vi "6517A.vi"() -> ()   [LabVIEW 2019]
uses:
  lib/Keithley 622x/Configure/Delta PDelta DCon Modes/Low Level/Typedefs/KE622x -- Delta DCon Mode Delay.ctl
  <vilib>/Utility/file.llb/Write Delimited Spreadsheet (DBL).vi
  lib/Keithley 622x/Keithley 622x.lvlib
  lib/Keithley 6517/Keithley 6517.lvlib
panel:
  in  "I(A)":dbl
  out "XY图":cluster{dbl[], dbl[]}(graph)
  in  "file path (dialog if empty)":path caption="文件路径 （空时为对话框）"
  in  "622x Resource":refnum<visa-resource-name>
  in  "Meas Timeout\n(msecs)":u32=20000
  out "Execution Time\n(secs)":dbl
  in  "Instrument Type":i32(ring)=3 items=["PPMS", "VersaLab", "DynaCool", "SVSM"]
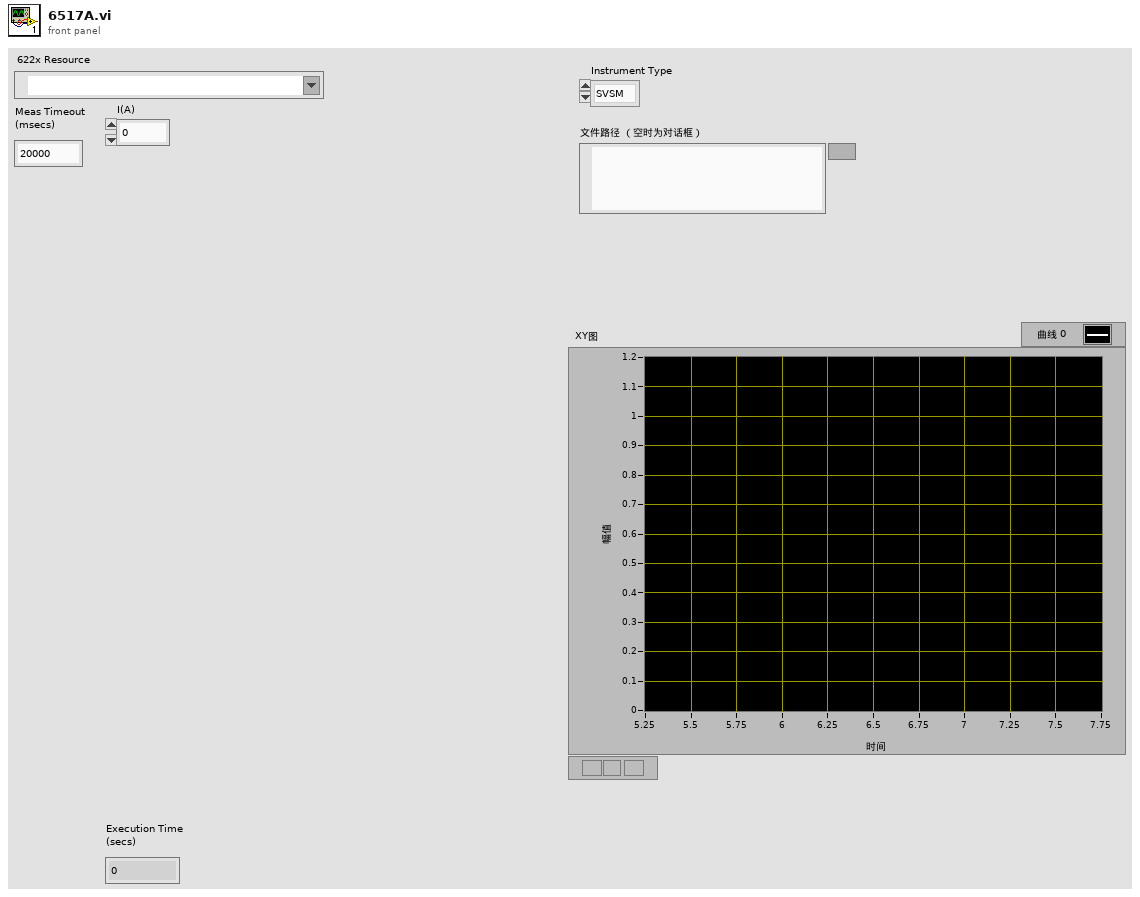
[diagram p1: front panel]
types:
  T1 = enum16{"open", "replace", "create", "open or create", "replace or create", "replace or create with confirmation"}
  T2 = typedef "Keithley 622x.lvlib/KE622x -- Delta DCon Mode Delay.ctl" = dbl
  T3 = cluster{"Measurement":dbl, "Units":string, "Time Stamp and Date":string, "Reading #":dbl, "Channel #":dbl}
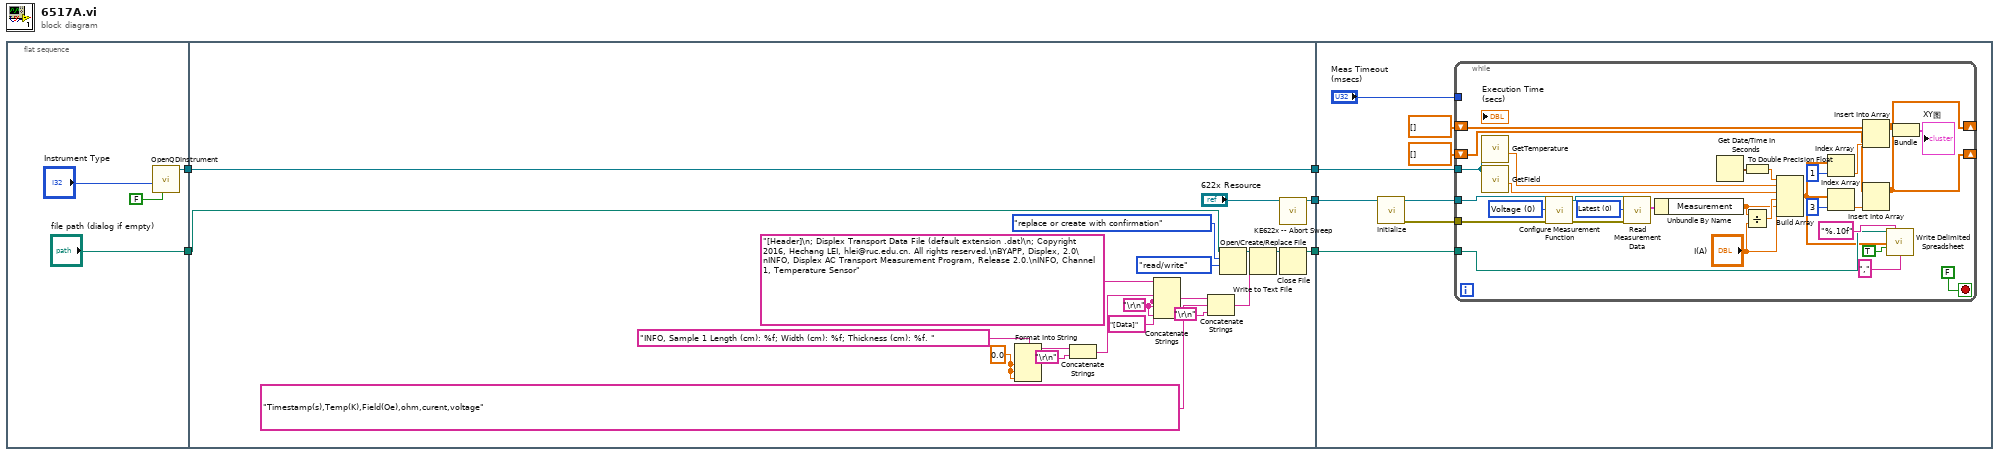
[diagram p0: block diagram]
diagram:
  n1 = flat-sequence {
    tunnel: [w7] -> w5
    tunnel: ["file path (dialog if empty)"] -> w3
    tunnel: w5 -> [w30]
    tunnel: [w30] -> w4
    tunnel: w3 -> [w18]
    tunnel: [w13] -> w2
    tunnel: [w10] -> w1
    tunnel: w4 -> [w38]
    tunnel: w2 -> [w36]
    tunnel: w1 -> [w33]
    frame #0 {
      n2 = call "OpenQDInstrument.vi"("Remote"=FALSE, "Instrument Type"="Instrument Type") -> ("Instrument Ref"=w7:refnum<k24>)  [unwired: 6 in, 1 out]
    }
    frame #1 {
      w25 = 0.0 ("输入 1")
      w22 = "\r\n"
      n3 = Format Into String(format string="INFO, Sample 1 Length (cm): %f; Width (cm): %f; Thickness (cm): %f. " ("string"), w25, w25, w25) -> (resulting string=w27:string)  [unwired: 2 in, 1 out]
      n4 = Concatenate Strings(w27, "\r\n") -> (w29:string)
      n5 = Concatenate Strings("[Header]\n; Displex Transport Data File (default extension .dat)\n; Copyright 2016, Hechang LEI, hlei@ruc.edu.cn. All rights reserved.\nBYAPP, Displex, 2.0\nINFO, Displex AC Transport Measurement Program, Release 2.0.\nINFO, Channel 1, Temperature Sensor" ("string"), w22, w29, w22, "[Data]" ("string"), w22) -> (w28:string)
      n6 = Concatenate Strings(w28, "Timestamp(s),Temp(K),Field(Oe),ohm,curent,voltage" ("字符串"), "\r\n") -> (w19:string)
      n7 = Open/Create/Replace File(file path (use dialog)=w18, operation (0:open)=T1."replace or create with confirmation" ("操作(0:open)"), access (0:read/write)=enum16{"read/write", "read-only", "write-only"}."read/write" ("权限(0:read/write)")) -> (refnum out=w17:refnum<file>)  [unwired: 3 in, 2 out]
      n8 = Write to Text File(file (use dialog)=w17, text=w19) -> (refnum out=w14:refnum<file>)  [unwired: 2 in, 2 out]
      n9 = call "KE622x -- Abort Sweep.vi"("Resource In"="622x Resource") -> ("Resource Out (dupl)"=w10:refnum<visa-resource-name>)  [unwired: 13 in, 1 out]
      n10 = Close File(refnum=w14) -> (path=w13:path)  [unwired: 1 in, 1 out]
    }
    frame #2 {
      n11 = call "Initialize.vi"("VISA resource name"=w33) -> ("error out"=w31:errorcluster, "VISA resource name out"=w32:refnum<visa-resource-name>)  [unwired: 9 in]
      n12 = while {
        tunnel: w38 -> [w67]
        tunnel: "Meas Timeout\n(msecs)" -> [_]
        tunnel: w36 -> [w62]
        shift-right: [w51] -> _
        shift-left: T2[] [] -> [w54]
        shift-right: [w52] -> _
        shift-left: T2[] [] -> [w56]
        tunnel: w32 -> [w46]
        tunnel: w31 -> [w43]
        stop <- FALSE stop-if-true
        w45 = 0 items=["Voltage", "Current", "Resistance", "Charge"] ("Measurement Function (0: Voltage)")
        w48 = 0 items=["Latest", "New"] ("Reading Option (0: Latest)")
        n13 = call "GetTemperature.vi"("Instrument Ref In"=w67) -> ("Temperature"=w66:dbl)  [unwired: 4 in, 4 out]
        n14 = call "GetField.vi"("Instrument Ref In"=w67) -> ("Field"=w65:dbl)  [unwired: 4 in, 4 out]
        n15 = call "Configure Measurement Function.vi"("error in (no error)"=w43, "Measurement Function (0: Voltage)"=w45, "VISA resource name"=w46) -> ("error out"=w42:errorcluster, "VISA resource name out"=w44:refnum<visa-resource-name>)  [unwired: 7 in]
        n16 = call "Read Measurement Data.vi"("error in (no error)"=w42, "Reading Option (0: Latest)"=w48, "VISA resource name"=w44) -> ("Measurement"=w47:T3)  [unwired: 6 in, 2 out]
        n17 = Unbundle By Name(w47) -> ("Measurement"=w40:dbl)
        n18 = Get Date/Time In Seconds() -> (seconds since 1Jan1904=w61:timestamp)
        n19 = Divide(x=w40, y="I(A)") -> (x/y=w41:dbl)
        n20 = To Double Precision Float(number=w61) -> (double precision float=w60:dbl)
        n21 = Build Array(w60, w66, w65, w41, w40, "I(A)") -> (w57:dbl[])
        n22 = Index Array(array=w57, index=1 ("索引")) -> (element=w55:dbl)
        n23 = Index Array(array=w57, index=3 ("索引")) -> (element=w53:dbl)
        n24 = Insert Into Array(array=w56, new element=w55) -> (w52:T2[])  [unwired: 1 in]
        n25 = Insert Into Array(array=w54, new element=w53) -> (w51:T2[])  [unwired: 1 in]
        n26 = call-poly <vilib>:"Write Delimited Spreadsheet.vi"("file path (dialog if empty)"=w62, "format (%.3f)"="%.10f", "1D data"=w57, "append to file? (new file:F)"=TRUE, "delimiter (\\t)"="," ("delimiter (\\t)")) -> ()  [unwired: 9 in, 2 out]
        n27 = Bundle(w52, w51) -> (→"XY图":cluster{T2[], T2[]})  [unwired: 1 in]
      }
    }
  }
